vi "Maui 2.0. Set Subpanels.Path Array.vi"(6 "Append (F)":bool, 8 "error in (no error)":errorcluster, 10 "Subpanel List":path[](array[path]), 11 "Maui 2.0 in":refnum<class "Maui 2.0.lvclass">) -> (0 "error out":errorcluster, 2 "Subpanels":refnum<class "SMO.lvclass">[](array[class]), 3 "Maui 2.0 out":refnum<class "Maui 2.0.lvclass">)   [LabVIEW 2019, in "Maui 2.0.lvclass"]
uses:
  Maui 2.0.lvclass
  <vilib>/JKI/JKI SMO/SMO/SMO.lvclass
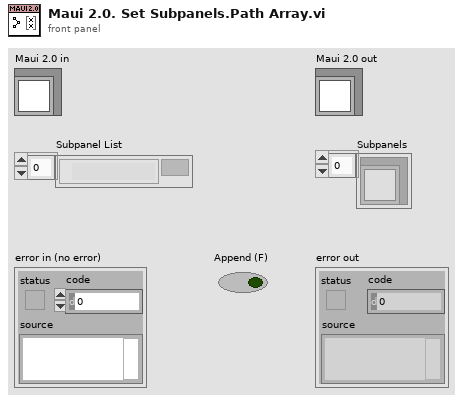
[diagram p1: front panel]
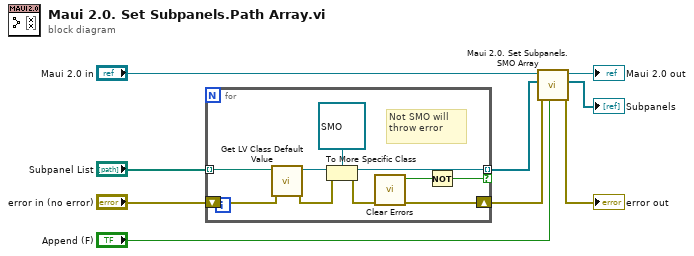
[diagram p0: block diagram]
diagram:
  n1 = for {
    tunnel: "Subpanel List" -> [w19] mode=indexing
    shift-right: [w15] -> w3
    shift-left: "error in (no error)" -> [w12]
    tunnel: [w14] -> w5 mode=indexing if=w10
    # "Not SMO will throw error"
    n2 = call <vilib>:"Get LV Class Default Value.vi"("error in (no error)"=w12, "class path"=w19) -> ("error out"=w11:errorcluster, "object"=w18:refnum<class>)  [unwired: 8 in]
    n3 = To More Specific Class(target class=refnum<class "SMO.lvclass"> refnum ("SMO"), reference=w18, error in=w11) -> (specific class reference=w14:refnum<class "SMO.lvclass">, error out=w16:errorcluster)
    n4 = call <vilib>:"Clear Errors.vi"("error in (no error)"=w16) -> ("error out"=w15:errorcluster, "specific error cleared?"=w13:bool)  [unwired: 5 in]
    n5 = Not(x=w13) -> (.not. x?=w10:bool)
  }
  n6 = call-dynamic "Maui 2.0. Set Subpanels.SMO Array.vi"("Append (F)"="Append (F)", "error in (no error)"=w3, "Subpanels in"=w5, "Maui 2.0 in"="Maui 2.0 in") -> ("error out"=→"error out":errorcluster, "Subpanels Out"=→"Subpanels":refnum<class "SMO.lvclass">[], "Maui 2.0 out"=→"Maui 2.0 out":refnum<class "Maui 2.0.lvclass">)  [unwired: 5 in]
